vi "enumerateStaticDependencies.vi"(8 "error in (no error)":errorcluster, 11 "Instrument.Lockin":refnum<class "Instrument.Lockin.lvclass">) -> (0 "error out":errorcluster, 2 "Static Dependencies":refnum<class "Dependency.lvclass">[](array[class]), 3 "Instrument.Lockin out":refnum<class "Instrument.Lockin.lvclass">)   [LabVIEW 2019, in "Instrument.Lockin.lvlib" / "Instrument.Lockin.lvclass"]
doc: "JKI State Machine Objects (SMO) 1.3.0.56\nJKI - JKI\nCopyright (c) 2017, JKI"
uses:
  Instrument.Lockin.lvclass
  <vilib>/JKI/JKI SMO/Dependency/Dependency.lvclass
  Instrument.Lockin.lvclass/Instrument.Lockin.ctl
  Instrument.DAQ/Instrument.DAQ.lvclass
  C:/Program Files/National Instruments/LabVIEW 2019/vi.lib/JKI/JKI SMO/SMO/SMO.lvclass
  <userlib>/LevyLab/Instrument Framework/Instrument Types/Lockin/Instrument.LockinAPI.lvclass
  <vilib>/JKI/JKI SMO/SMO/SMO.lvclass
panel:
  # "For instructions on how to use the JKI State Machine Objects, examples and video tutorials, visit:\nhttp://jki.net/state-machine-objects/\n\nJKI State Machine Objects™\nhttp://jki.net/state-machine-objects/\nCopyright (C) 2005-2015, JKI <info@jki.net>\nALL RIGHTS RESERVED"
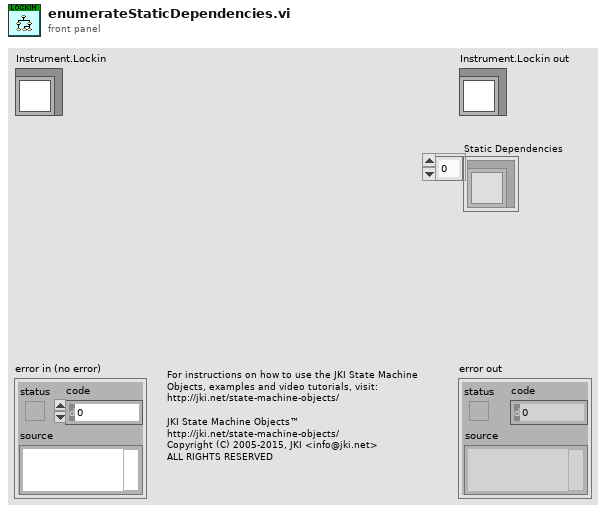
[diagram p1: front panel]
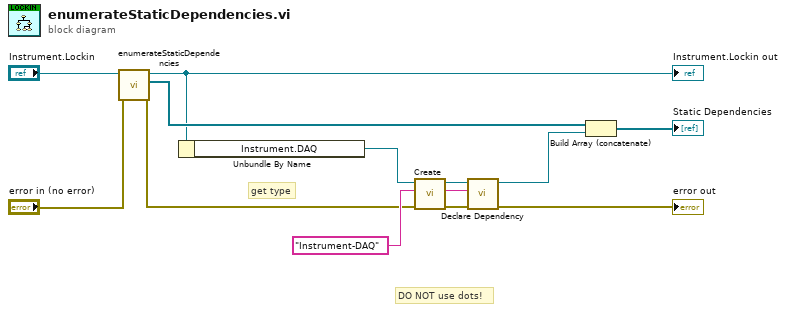
[diagram p0: block diagram]
diagram:
  # "get type"
  # "DO NOT use dots!"
  n1 = call-parent "enumerateStaticDependencies.vi"("error in (no error)"="error in (no error)", "Instrument"="Instrument.Lockin") -> ("error out"=w10:errorcluster, "Static Dependencies"=w9:refnum<class "Dependency.lvclass">[], "Instrument out"=w6:refnum<class "Instrument.Lockin.lvclass">)  [unwired: 7 in]
  "Instrument.Lockin out" <- w6
  n2 = Unbundle By Name(w6) -> ("Instrument.DAQ"=w8:refnum<class "Instrument.DAQ.lvclass">)
  n3 = call <vilib>:"Create.vi"("error in (no error)"=w10, "Subsystem Name (optional)"="Instrument-DAQ" ("Name"), "SMO"=w8) -> ("error out"=w4:errorcluster, "SMO name"=w3:string, "SMO out"=w5:refnum<class "Instrument.DAQ.lvclass">)  [unwired: 6 in]
  n4 = call <vilib>:"Declare Dependency.vi"("error in (no error)"=w4, "Name"=w3, "Type"=w5) -> ("error out"=→"error out":errorcluster, "Dependency out"=w2:refnum<class "Dependency.lvclass">)  [unwired: 7 in]
  n5 = Build Array (concatenate)(w9, w2) -> (→"Static Dependencies":refnum<class "Dependency.lvclass">[])
